vi "AssertControlVisible_Tests.vi"(8 "error in (no error)":errorcluster) -> (0 "error out":errorcluster)   [LabVIEW 2016, in "DronaTest.lvlib"]
uses:
  DronaTest.lvlib
  APIs/Stimulus/ControlValue/ValueSignalByPathString.vi
  APIs/Assert/AssertControlVisible/AssertVisible.vi
  APIs/Assert/AssertControlVisible/AssertInvisible.vi
  Drona.lvlib
  <vilib>/addons/_JKI Toolkits/Caraya/classes/Assert/Assert.lvclass
  AssertControlVisible.lvlib
  <vilib>/addons/_JKI Toolkits/Caraya/classes/Test/Test.lvclass
  APIs/Stimulus/ControlValue/ControlValue.lvlib
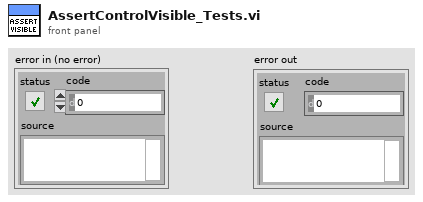
[diagram p1: front panel]
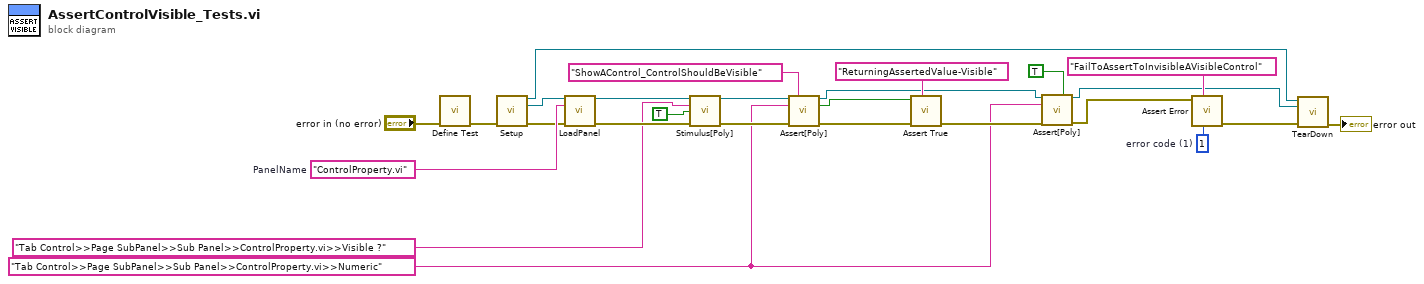
[diagram p0: block diagram]
diagram:
  w6 = 1  # error code (1)
  w1 = "Tab Control>>Page SubPanel>>Sub Panel>>ControlProperty.vi>>Numeric" ("Control Path")
  w25 = "ControlProperty.vi"  # PanelName
  n1 = call <vilib>:"Define Test.vi"("error in (no error)"="error in (no error)") -> ("error out"=w19:errorcluster)  [unwired: 9 in, 1 out]
  n2 = call "Setup.vi"("error in (no error)"=w19) -> ("Application Ref"=w15:refnum<vi>, "VI out"=w20:refnum<vi>, "error out"=w21:errorcluster)  [unwired: 12 in]
  n3 = call "LoadPanel.vi"("VI in"=w20, "Panel Name"=w25, "error in (no error)"=w21) -> ("VI out"=w12:refnum<vi>, "error out"=w22:errorcluster)  [unwired: 11 in]
  n4 = call-poly "Stimulus[Poly].vi"("VI Reference In"=w12, "Control Path"="Tab Control>>Page SubPanel>>Sub Panel>>ControlProperty.vi>>Visible ?", "Value (Signaling)"=TRUE, "error in"=w22) -> ("VI Reference Out"=w24:refnum<vi>, "error out"=w14:errorcluster)  [unwired: 10 in]
  n5 = call-poly "Assert[Poly].vi"("VI Reference In"=w24, "Label"="ShowAControl_ControlShouldBeVisible" ("string"), "Control Path"=w1, "Error In"=w14) -> ("VI Reference Out"=w5:refnum<vi>, "Asserted Value"=w13:bool, "Error Out"=w17:errorcluster)  [unwired: 9 in]
  n6 = call <vilib>:"Assert True.vi"("Label"="ReturningAssertedValue-Visible", "error in (no error)"=w17, "True?"=w13) -> ("error out"=w3:errorcluster)  [unwired: 7 in, 1 out]
  n7 = call-poly "Assert[Poly].vi"("VI Reference In"=w5, "Assert Only? (F)"=TRUE, "Control Path"=w1, "Error In"=w3) -> ("VI Reference Out"=w4:refnum<vi>, "Error Out"=w9:errorcluster)  [unwired: 9 in, 1 out]
  n8 = call <vilib>:"Assert Error.vi"("error code (1)"=w6, "Label"="FailToAssertToInvisibleAVisibleControl", "Error?"=w9) -> ("error out"=w2:errorcluster)  [unwired: 7 in, 1 out]
  n9 = call "TearDown.vi"("Application Ref"=w15, "VI in"=w4, "error in (no error)"=w2) -> ("error out"=→"error out":errorcluster)  [unwired: 12 in]
